vi "_Parse Detected Modulation List.vi"(8 "error in (no error)":errorcluster, 10 "Input String":string, 11 "VISA resource name":refnum<visa-resource-name>) -> (0 "error out":errorcluster, 1 "Detected Modulations":i32[](array[numeric]), 2 "Reliability":i32, 3 "VISA resource name out":refnum<visa-resource-name>)   [LabVIEW 2020, in "Rohde&Schwarz CMWXP NR FR1 Measurement.lvlib"]
uses:
  <instrlib>/Rohde&Schwarz CMWXP NR FR1 Measurement/Rohde&Schwarz CMWXP NR FR1 Measurement.lvlib
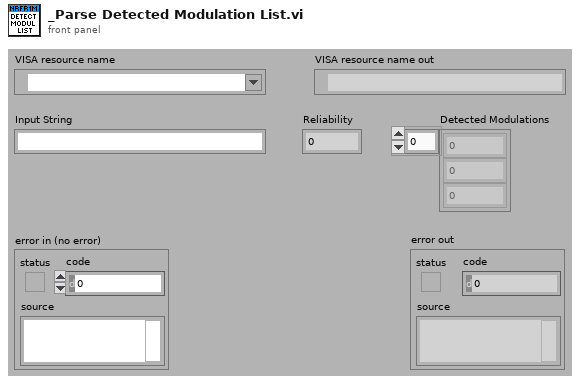
[diagram p1: front panel]
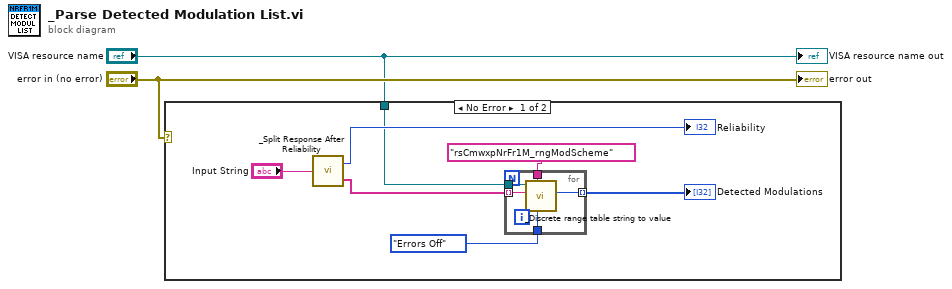
[diagram p0: block diagram]
diagram:
  n1 = case shown="No Error" "error in (no error)" {
    tunnel: "VISA resource name" -> [w3 _]
    frame No Error {
      n2 = call <instrlib>:"_Split Response After Reliability.vi"("Input String"="Input String") -> ("Response out"=w6:string[], "Reliability out"=→"Reliability":i32)
      n3 = for {
        tunnel: "rsCmwxpNrFr1M_rngModScheme" -> [w14]
        tunnel: [w13] -> w5 mode=indexing
        tunnel: w6 -> [w12] mode=indexing
        tunnel: enum16{"Errors Off", "Errors", "Warnings"}."Errors Off" ("Error Mode (Warnings)") -> [w11]
        tunnel: w3 -> [w10]
        n4 = call <instrlib>:"_Discrete range table string to value.vi"("Error Mode (Warnings)"=w11, "Discrete Range Table Identifier"=w14, "String Value In"=w12, "VISA resource name"=w10) -> ("Enum Value"=w13:i32)  [unwired: 5 in, 2 out]
      }
      "Detected Modulations" <- w5
    }
    frame Error {
    }
  }
  "VISA resource name out" <- "VISA resource name"
  "error out" <- "error in (no error)"
